vi "Coherence Length.vi"() -> ()   [LabVIEW 2017]
uses:
  <vilib>/Platform/TimedLoop/XDataNode/timing_clust.ctl
  <vilib>/Platform/TimedLoop/XDataNode/nitl_modes.ctl
  <vilib>/Platform/TimedLoop/XDataNode/wakeup.ctl
  <vilib>/gmath/NumericalOptimization/Nonlinear Curve Fit LM formula string.vi
  <vilib>/Utility/file.llb/Write Delimited Spreadsheet (I64).vi
  <vilib>/platform/TimedLoop/XDataNode/XDataNode.xnode
  <vilib>/gmath/NI_Gmath.lvlib
  <vilib>/Platform/TimedLoop/XDataNode/XDNodeRunTimeDep.lvlib
  <vilib>/Analysis/NI_AALBase.lvlib
panel:
  out "Waveform Chart":dynamicdata(graph)
  in  "Position":string
  in  "base path":path
  in  "Profiles X 2":refnum<k7>(container)
  out "best fit parameters 2":dbl[](array[numeric])
  out "Far camera":dynamicdata(graph)
  out "best fit parameters":dbl[](array[numeric])
  in  "length":i32=800
  out "Near Camera":dynamicdata(graph)
  in  "Yg 2":refnum<k7>(container)
  in  "Xg 2":refnum<k7>(container)
  in  "Yc 2":refnum<k7>(container)
  in  "Xc 2":refnum<k7>(container)
  out "Exposure 2":refnum<k7>(container)
  in  "Mean 2":refnum<k7>(container)
  in  "Profiles Y 2":refnum<k7>(container)
  in  "Minor 2":refnum<k7>(container)
  in  "PaletteBar 2":refnum<k7>(container)
  in  "Major 2":refnum<k7>(container)
  in  "CCDimage 2":refnum<k7>(container)
  in  "Yg 1":refnum<k7>(container)
  in  "Xg 1":refnum<k7>(container)
  in  "Yc 1":refnum<k7>(container)
  in  "Xc 1":refnum<k7>(container)
  in  "Exposure 1":refnum<k7>(container)
  in  "Mean 1":refnum<k7>(container)
  in  "Profiles Y1":refnum<k7>(container)
  in  "Minor 1":refnum<k7>(container)
  in  "Profiles X 1":refnum<k7>(container)
  in  "PaletteBar 1":refnum<k7>(container)
  in  "GetData":refnum<k7>(container)
  in  "Major 1":refnum<k7>(container)
  in  "CCDimage 1":refnum<k7>(container)
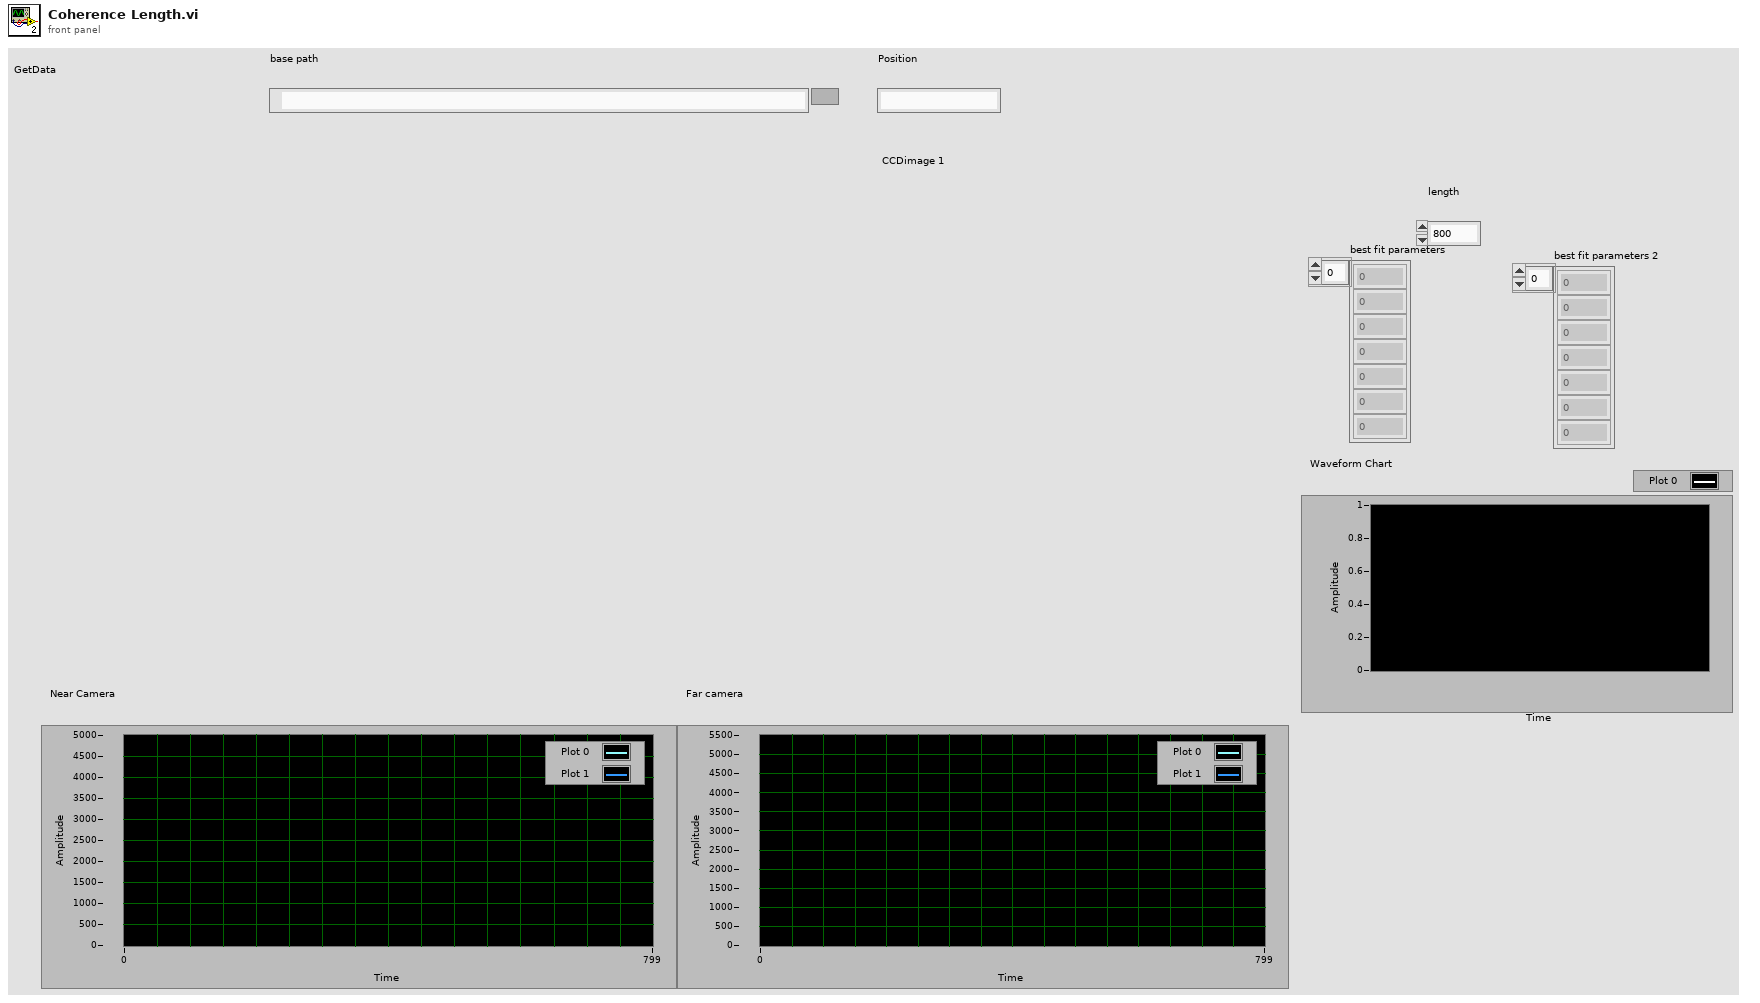
[diagram p1: front panel]
types:
  T1 = typedef "XDNodeRunTimeDep.lvlib/timing_clust.ctl" = cluster{"Expected End [f-1]":u64, "Actual End [f-1]":u64, "Finished Late? [f-1]":bool, "Expected End [i-1]":u64, "Actual End [i-1]":u64, "Finished Late? [i-1]":bool, "Expected Start [i]":u64, "Actual Start [i]":u64, "Expected Start [f]":u64, "Actual Start [f]":u64, "Source Name":string, "Structure Name":string, "Period":i64, "Deadline":i64, "Offset":i64, "Start":i64, "Priority":i32, "Timeout":i32, "Mode":T2, "Wakeup Reason":T3, "Error":errorcluster, "Source Type":string, "Secondary Source Type":string, "Global End Time":u64, "Global Start Time":u64, "Frame Duration":u64, "Iteration Duration":u64, "Assigned CPU":i32, "I/O Scan Engine Mode":u32}
  T2 = typedef "XDNodeRunTimeDep.lvlib/nitl_modes.ctl" = enum32{"No Change", "Process missed periods, maintain original phase", "Discard missed periods, maintain original phase", "Process missed periods, ignore original phase", "Discard missed periods, ignore original phase"}
  T3 = typedef "XDNodeRunTimeDep.lvlib/wakeup.ctl" = enum32{"Normal", "Aborted", "Asynchronous wakeup", "Timing source error", "Timed loop error", "Timeout"}
  T4 = cluster{"model":string, "Parameters":string[], "x":string}
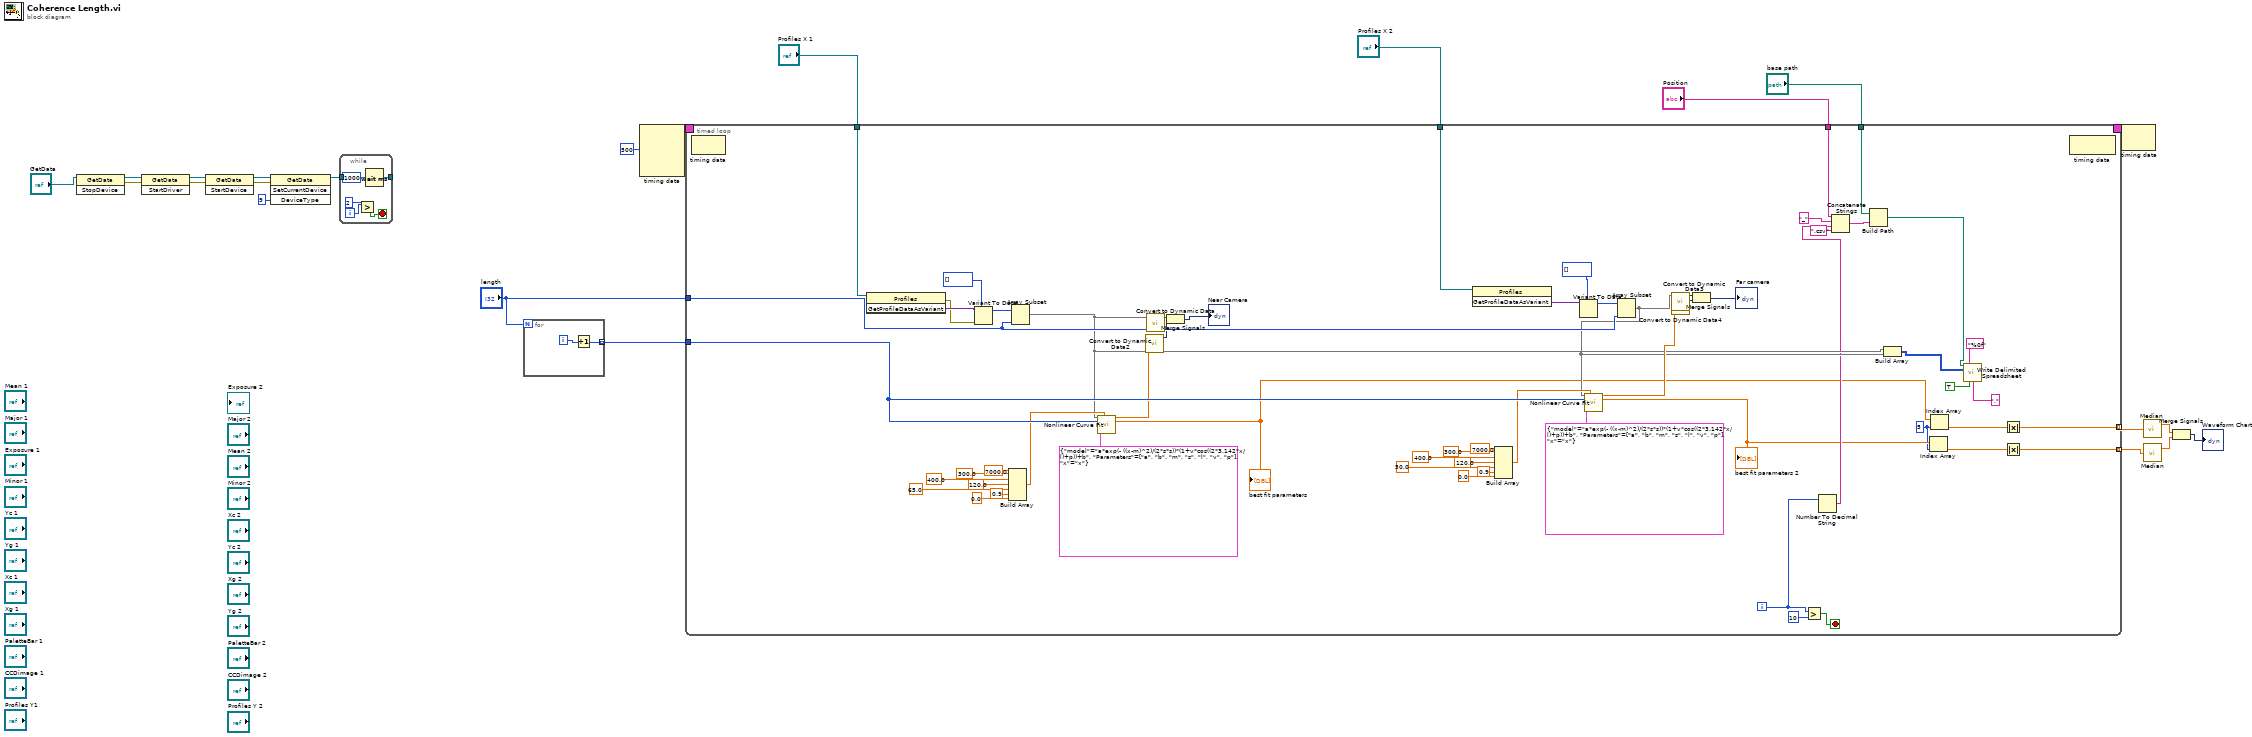
[diagram p0: block diagram]
diagram:
  n1 = invoke class="GetData" method="StopDevice"(reference="GetData") -> (reference out=w22:refnum<k7>, error out=w21:errorcluster)  [unwired: 2 in, 1 out]
  n2 = invoke class="GetData" method="StartDriver"(reference=w22, error in=w21) -> (reference out=w20:refnum<k7>, error out=w19:errorcluster)  [unwired: 1 in, 1 out]
  n3 = invoke class="GetData" method="StartDevice"(reference=w20, error in=w19) -> (reference out=w18:refnum<k7>, error out=w17:errorcluster)  [unwired: 1 in, 1 out]
  n4 = invoke class="GetData" method="SetCurrentDevice"(reference=w18, error in=w17, "DeviceType"=i16 9) -> (reference out=w15:refnum<k7>)  [unwired: 1 in, 3 out]
  n5 = while {
    tunnel: [w28] -> _
    tunnel: w15 -> [_]
    tunnel: w15 -> [w28]
    i -> [w26]
    stop <- w24 stop-if-true
    n6 = Greater?(x=w26, y=2) -> (0:w24:bool)
    n7 = Wait (ms)(milliseconds to wait=u32 1000) -> ()  [unwired: 1 out]
  }
  n8 = for {
    N: "length" -> [_]
    tunnel: [w29] -> w13 mode=indexing
    i -> [w30]
    n9 = Increment(x=w30) -> (x+1=w29:i32)
  }
  n10 = node-c288(i64 500 ("Period")) -> (w10:T1)  [unwired: 3 in]
  n11 = timed-loop {
    timing: w10 -> [_]
    timing-out: [_] -> w9
    tunnel: "length" -> [w90]
    tunnel: w13 -> [w89]
    tunnel: "Profiles X 1" -> [w88]
    tunnel: "Profiles X 2" -> [w54]
    tunnel: "base path" -> [w43]
    tunnel: "Position" -> [w42]
    tunnel: [w36] -> w5 mode=indexing
    tunnel: [w35] -> w4 mode=indexing
    i -> [w48]
    stop <- w52 stop-if-true
    w39 = 5 ("index")
    n12 = node-c288() -> ()  [unwired: 1 in, 1 out]
    n13 = invoke class="Profiles" method="GetProfileDataAsVariant"(reference=w88) -> (error out=w55:errorcluster, "GetProfileDataAsVariant"=w87:variant)  [unwired: 2 in, 1 out]
    n14 = Variant To Data(error in=w55, type=i32[] [], Variant=w87) -> (data=w86:i32[])  [unwired: 1 out]
    n15 = Build Array(7000.0 ("element"), 300.0 ("element"), 400.0 ("element"), 120.0 ("element"), 65.0 ("element"), 0.9 ("element"), 0.0 ("element")) -> (w76:dbl[])
    n16 = Array Subset(array=w86, length=w90) -> (w51:i32[])  [unwired: 1 in]
    n17 = call-poly <vilib>:"Nonlinear Curve Fit.vi"("Y"=w51, "initial parameters"=w76, "X"=w89, "model description"=T4 {"model"="a*exp(- ((x-m)^2)/(2*s*s))*(1+v*cos((2*3.142*x/l)+p))+b", "Parameters"=["a", "b", "m", "s", "l", "v", "p"], "x"="x"}) -> ("best nonlinear fit"=w74:dbl[], "best fit parameters"=w40:dbl[])  [unwired: 7 in, 3 out]
    "best fit parameters" <- w40
    n18 = call "Convert to Dynamic Data2"("Array"=w74) -> ("Dynamic Data Type"=w73:dynamicdata)  [unwired: 3 in]
    n19 = call "Convert to Dynamic Data"("Array"=w51) -> ("Dynamic Data Type"=w75:dynamicdata)  [unwired: 3 in]
    n20 = Merge Signals(w75, w73) -> (→"Near Camera":dynamicdata)
    n21 = invoke class="Profiles" method="GetProfileDataAsVariant"(reference=w54) -> ("GetProfileDataAsVariant"=w71:variant)  [unwired: 2 in, 2 out]
    n22 = Build Array(7000.0 ("element"), 300.0 ("element"), 400.0 ("element"), 120.0 ("element"), 50.0 ("element"), 0.9 ("element"), 0.0 ("element")) -> (w62:dbl[])
    n23 = Variant To Data(type=i32[] [], Variant=w71) -> (data=w56:i32[])  [unwired: 1 in, 1 out]
    n24 = Array Subset(array=w56, length=w90) -> (w50:i32[])  [unwired: 1 in]
    n25 = call-poly <vilib>:"Nonlinear Curve Fit.vi"("Y"=w50, "initial parameters"=w62, "X"=w89, "model description"=T4 {"model"="a*exp(- ((x-m)^2)/(2*s*s))*(1+v*cos((2*3.142*x/l)+p))+b", "Parameters"=["a", "b", "m", "s", "l", "v", "p"], "x"="x"}) -> ("best nonlinear fit"=w59:dbl[], "best fit parameters"=w41:dbl[])  [unwired: 7 in, 3 out]
    "best fit parameters 2" <- w41
    n26 = call "Convert to Dynamic Data3"("Array"=w50) -> ("Dynamic Data Type"=w60:dynamicdata)  [unwired: 3 in]
    n27 = call "Convert to Dynamic Data4"("Array"=w59) -> ("Dynamic Data Type"=w58:dynamicdata)  [unwired: 3 in]
    n28 = Merge Signals(w60, w58) -> (→"Far camera":dynamicdata)
    n29 = Greater?(x=w48, y=10) -> (0:w52:bool)
    n30 = Number To Decimal String(number=w48) -> (decimal integer string=w47:string)  [unwired: 1 in]
    n31 = Concatenate Strings(w42, "_" ("string"), w47, ".csv" ("string")) -> (w44:string)
    n32 = Build Path(base path=w43, name or relative path=w44) -> (appended path=w49:path)
    n33 = Build Array(w51, w50) -> (w33:i32[][])
    n34 = Index Array(array=w41, index=w39) -> (element=w37:dbl)
    n35 = Index Array(array=w40, index=w39) -> (element=w38:dbl)
    n36 = call-poly <vilib>:"Write Delimited Spreadsheet.vi"("file path (dialog if empty)"=w49, "format (%d)"="%0f", "2D data"=w33, "transpose? (no:F)"=TRUE, "delimiter (\\t)"="," ("delimiter (\\t)")) -> ()  [unwired: 9 in, 2 out]
    n37 = Absolute Value(x=w38) -> (abs(x)=w36:dbl)
    n38 = Absolute Value(x=w37) -> (abs(x)=w35:dbl)
    n39 = node-c288() -> ()  [unwired: 1 in, 1 out]
  }
  n40 = node-c288(w9) -> ()  [unwired: 1 out]
  n41 = call <vilib>:"Median.vi"("X"=w5) -> ("median"=w3:dbl)  [unwired: 1 out]
  n42 = call <vilib>:"Median.vi"("X"=w4) -> ("median"=w2:dbl)  [unwired: 1 out]
  n43 = Merge Signals(w3, w2) -> (→"Waveform Chart":dynamicdata)
